vi "TomScan1762WithPumpingHWT.vi"() -> ()   [LabVIEW 2012]
uses:
  <vilib>/Utility/file.llb/Write To Spreadsheet File (DBL).vi
panel:
  out "OP Waveform":digitalwaveform(waveform)={"t0"=timestamp(0 s since 1904-01-01), "dt"=0.0, "Y"={"transitions"=[], "data"=[]}, "error"={"status"=FALSE, "code"=37421928, "source"=""}}
  in  "Comment":string="SPAOM, 3000 mA, 60 mA, 150 mA, now being mixed with 20 MHz, 7V Res, 89 MHz DPAOM"
  in  "B Field":dbl=3.0
  in  "Power":dbl=4.0
  out "digital waveform":digitalwaveform(waveform)={"t0"=timestamp(0 s since 1904-01-01), "dt"=0.001, "Y"={"transitions"=[], "data"=array3001x1[3001 elements]}}
  in  "Real Cutoff":dbl=26.0
  in  "Microseconds Expose":i32=300
  out "Shelving Events":dbl=11.0
  out "Dark Counts":dbl=19.0
  out "Bright Counts":dbl=61.0
  in  "Rerun BG":dbl=50.0
  in  "Interval":dbl=0.03
  in  "Runs for Background":dbl=50.0
  out "Average counts":dbl=59.98
  out "Cutoff":dbl=26.0
  in  "Cutoff Limit":dbl=10.0
  in  "OP Time":dbl=10.0
  in  "Op Pump":bool=TRUE
  in  "Runs per data point":dbl=100.0
  in  "Step Size":dbl(slide)=2000.0 min=100.0 max=100000.0 step=1.0 scale=100.0..100000.0 scale format="%#.0f"
  in  "Low Freq":dbl(slide)=78950000.0 min=50000000.0 max=120000000.0 step=1000.0 scale=50000000.0..120000000.0 scale format="%#.5f"
  in  "High Freq":dbl(slide)=79060000.0 min=50000000.0 max=120000000.0 step=1000.0 scale=50000000.0..120000000.0 scale format="%#.0f"
  out "Cur Freq":dbl=78998000.0 format="%#_8f"
  out "Path":path=path "c:/data/1762 Scans/2009-11-09_16-22-05_1762scanWithPumping.txt"
  out "Frequency Scan":cluster{dbl, dbl}[](graph)=[{79100000.0, 0.0}, {79098000.0, 0.01}, {79096000.0, 0.0}, {79094000.0, 0.0}, {79092000.0, 0.0}, {79090000.0, 0.01}, {79088000.0, 0.0}, {79086000.0, 0.0}, {79084000.0, 0.0}, {79082000.0, 0.0}, {79080000.0, 0.0}, {79078000.0, 0.0}, {79076000.0, 0.0}, {79074000.0, 0.02}, {79072000.0, 0.0}, {79070000.0, 0.0}, {79068000.0, 0.0}, {79066000.0, 0.0}, {79064000.0, 0.01}, {79062000.0, 0.0}, {79060000.0, 0.0}, {79058000.0, 0.02}, {79056000.0, 0.01}, {79054000.0, 0.01}, {79052000.0, 0.02}, {79050000.0, 0.01}, {79048000.0, 0.01}, {79046000.0, 0.05}, {79044000.0, 0.01}, {79042000.0, 0.01}, {79040000.0, 0.04}, {79038000.0, 0.02}, {79036000.0, 0.07}, {79034000.0, 0.07}, {79032000.0, 0.04}, {79030000.0, 0.08}, {79028000.0, 0.16}, {79026000.0, 0.22}, {79024000.0, 0.27}, {79022000.0, 0.31}, {79020000.0, 0.37}, {79018000.0, 0.49}, {79016000.0, 0.44}, {79014000.0, 0.36}, {79012000.0, 0.37}, {79010000.0, 0.48}, {79008000.0, 0.23}, {79006000.0, 0.29}, {79004000.0, 0.02}, {79002000.0, 0.02}, {79000000.0, 0.11}]
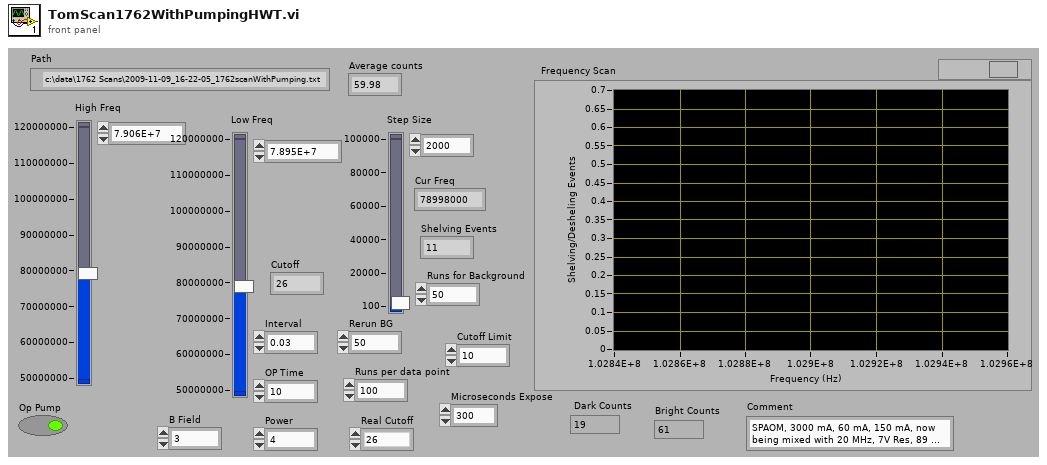
[diagram p1: front panel]
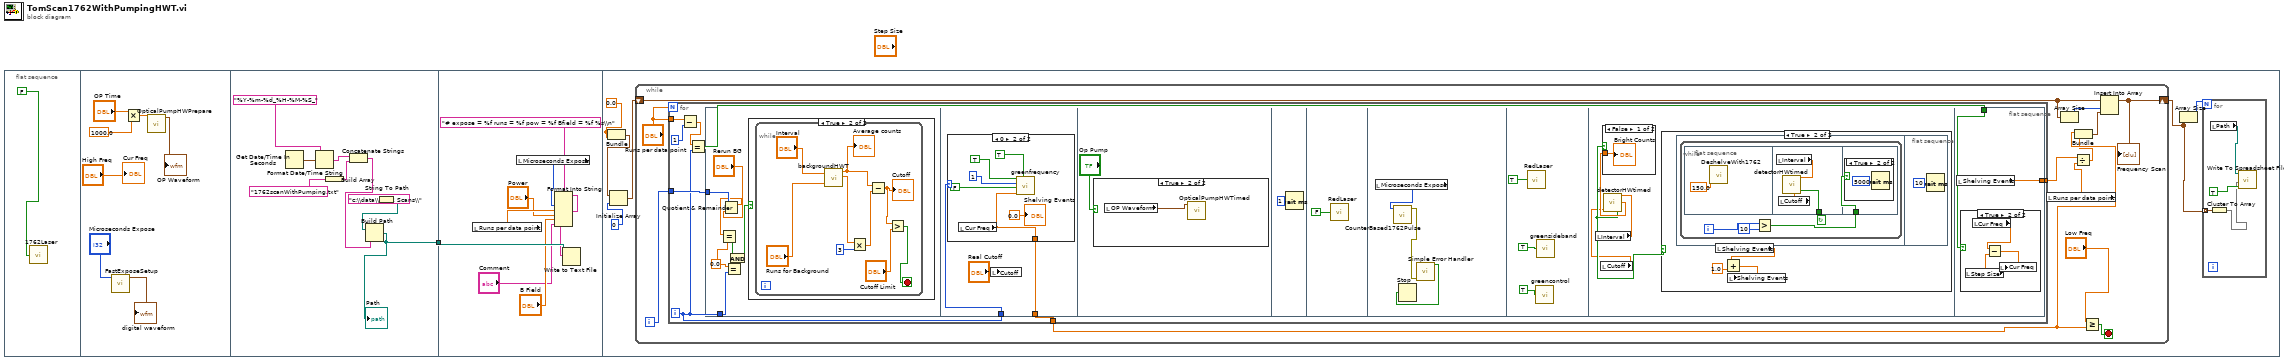
[diagram p0: block diagram]
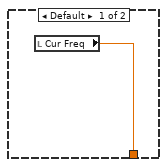
[diagram p3: hidden frame]
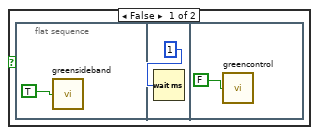
[diagram p4: hidden frame]
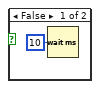
[diagram p6: hidden frame]
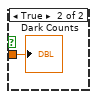
[diagram p7: hidden frame]
diagram:
  n1 = flat-sequence {
    tunnel: [w10] -> w1
    tunnel: w1 -> [w26]
    frame #0 {
      n2 = call "1762Laser.vi"("1762 Laser"=FALSE) -> ()
    }
    frame #1 {
      n3 = call "FastExposeSetup.vi"("Microseconds Expose"="Microseconds Expose") -> ("digital waveform"=→"digital waveform":digitalwaveform)  [unwired: 10 in]
      n4 = Multiply(x="OP Time", y=1000.0) -> (x*y=w4:dbl)
      n5 = call "OpticalPumpHWPrepare.vi"("Pump Expose Time (us)"=w4) -> ("digital waveform out"=→"OP Waveform":digitalwaveform)  [unwired: 8 in]
      "Cur Freq" <- "High Freq"
    }
    frame #2 {
      n6 = Get Date/Time In Seconds() -> (seconds since 1Jan1904=w12:timestamp)
      n7 = Format Date/Time String(time format string (%c)="%Y-%m-%d_%H-%M-%S_", seconds (now)=w12) -> (date/time string=w14:string)  [unwired: 1 in]
      n8 = Build Array("1762scanWithPumping.txt") -> (w17:string[])
      n9 = Concatenate Strings(w14, w17) -> (w16:string)
      n10 = String To Path(string="c:\\data\\1762 Scans\\") -> (path=w18:path)
      n11 = Build Path(base path=w18, name or relative path=w16) -> (appended path=w10:path)
      "Path" <- w10
    }
    frame #3 {
      n12 = local read "Runs per data point"() -> (w22:dbl)
      n13 = local read "Microseconds Expose"() -> (w23:i32)
      n14 = Format Into String(format string="# expose = %f runs = %f pow = %f Bfield = %f %s\\n", w23, w22, "Power", "B Field", "Comment") -> (resulting string=w24:string)  [unwired: 2 in, 1 out]
      n15 = Write to Text File(file (use dialog)=w26, text=w24) -> ()  [unwired: 2 in, 3 out]
    }
    frame #4 {
      w31 = 0.0
      n16 = Bundle(w31, w31) -> (w32:cluster{dbl, dbl})  [unwired: 1 in]
      n17 = Initialize Array(w32, 0) -> (w29:cluster{dbl, dbl}[])
      n18 = while {
        shift-right: [w40] -> w27
        shift-left: w29 -> [w41]
        i -> [w48]
        stop <- w46 stop-if-true
        n19 = for {
          N: "Runs per data point" -> [_]
          tunnel: w48 -> [w56]
          tunnel: [w55] -> w38
          tunnel: [w54] -> w45
          tunnel: "Runs per data point" -> [w49]
          i -> [w53]
          n20 = Subtract(x=w49, y=1) -> (x-y=w52:dbl)
          n21 = Equal?(x=w52, y=w53) -> (x = y?=w50:bool)
          n22 = flat-sequence {
            tunnel: w53 -> [w64]
            tunnel: w56 -> [w63]
            tunnel: w53 -> [w76]
            tunnel: [w75] -> w55
            tunnel: [w119] -> w54
            tunnel: w50 -> [w118]
            frame #0 {
              w60 = 0.0 ("x")
              n23 = Quotient & Remainder(x=w63, y="Rerun BG") -> (x-y*floor(x/y)=w61:dbl)  [unwired: 1 out]
              n24 = Equal?(x=w61, y=w60) -> (x = y?=w58:bool)
              n25 = Equal?(x=w60, y=w64) -> (x = y?=w59:bool)
              n26 = And(x=w58, y=w59) -> (x .and. y?=w57:bool)
              n27 = case shown="True" w57 {
                frame False {
                }
                frame True {
                  n28 = while {
                    stop <- w65 stop-if-true
                    n29 = call "backgroundHWT.vi"("Interval"="Interval", "Runs"="Runs for Background") -> ("Mean"=w72:dbl, "Deviation"=w71:dbl)  [unwired: 2 out]
                    "Average counts" <- w72
                    n30 = Multiply(x=w71, y=3) -> (x*y=w73:dbl)
                    n31 = Subtract(x=w72, y=w73) -> (x-y=w67:dbl)
                    "Cutoff" <- w67
                    n32 = Greater?(x=w67, y="Cutoff Limit") -> (0:w65:bool)
                  }
                }
              }
            }
            frame #1 {
              n33 = case shown="0" w76 {
                tunnel: [w77 w79] -> w75
                frame Default {
                  n34 = local read "Cur Freq"() -> (w77:dbl)
                }
                frame 0 {
                  n35 = local read "Cur Freq"() -> (w79:dbl)
                  n36 = call "greenfrequency.vi"("Send Frequency"=TRUE, "Level"=1, "Send Level"=FALSE, "Frequency"=w79, "Stop"=TRUE) -> ()  [unwired: 2 in]
                  "Shelving Events" <- 0.0 ("Shelving Events")
                }
              }
              n37 = local write "Cutoff"("Real Cutoff") -> ()
            }
            frame #2 {
              n38 = case shown="True" "Op Pump" {
                frame False {
                  n39 = flat-sequence {
                    frame #0 {
                      n40 = call "greensideband.vi"("Sideband On/Off"=TRUE) -> ()
                    }
                    frame #1 {
                      n41 = Wait (ms)(milliseconds to wait=1) -> ()  [unwired: 1 out]
                    }
                    frame #2 {
                      n42 = call "greencontrol.vi"("Green"=FALSE) -> ()
                    }
                  }
                }
                frame True {
                  n43 = local read "OP Waveform"() -> (w88:digitalwaveform)
                  n44 = call "OpticalPumpHWTimed.vi"("OP Waveform"=w88) -> ()  [unwired: 10 in, 1 out]
                }
              }
            }
            frame #3 {
              n45 = Wait (ms)(milliseconds to wait=u32 1) -> ()  [unwired: 1 out]
            }
            frame #4 {
              n46 = call "RedLaser.vi"("Red Laser"=FALSE) -> ()
            }
            frame #5 {
              n47 = local read "Microseconds Expose"() -> (w91:i32)
              n48 = call "CounterBased1762Pulse.vi"("High Time (us)"=w91) -> ("error out"=w92:errorcluster)  [unwired: 10 in]
              n49 = call <vilib>:"Simple Error Handler.vi"("error in (no error)"=w92) -> ("error?"=w93:bool)  [unwired: 4 in, 4 out]
              n50 = Stop(stop? (T)=w93) -> ()
            }
            frame #6 {
              n51 = call "RedLaser.vi"("Red Laser"=TRUE) -> ()
              n52 = call "greencontrol.vi"("Green"=TRUE) -> ()
              n53 = call "greensideband.vi"("Sideband On/Off"=TRUE) -> ()
            }
            frame #7 {
              n54 = local read "Interval"() -> (w99:dbl)
              n55 = local read "Cutoff"() -> (w97:dbl)
              n56 = call "detectorHWtimed.vi"("Cutoff"=w97, "Interval"=w99) -> ("Boolean"=w98:bool, "Counts"=w100:dbl)  [unwired: 3 in]
              n57 = case shown="False" w98 {
                tunnel: w100 -> [w116 w117]
                frame False {
                  "Bright Counts" <- w116
                }
                frame True {
                  "Dark Counts" <- w117
                }
              }
              n58 = case shown="True" w98 {
                frame False {
                }
                frame True {
                  n59 = flat-sequence {
                    frame #0 {
                      n60 = while {
                        i -> [w106]
                        stop <- w107 continue-if-true
                        n61 = flat-sequence {
                          tunnel: [w109] -> w107
                          tunnel: w104 -> [w112]
                          frame #0 {
                            n62 = call "DeshelveWith1762.vi"("Expose Time"=150.0) -> ()
                          }
                          frame #1 {
                            n63 = local read "Interval"() -> (w111:dbl)
                            n64 = local read "Cutoff"() -> (w110:dbl)
                            n65 = call "detectorHWtimed.vi"("Cutoff"=w110, "Interval"=w111) -> ("Boolean"=w109:bool)  [unwired: 3 in, 1 out]
                          }
                          frame #2 {
                            n66 = case shown="True" w112 {
                              frame False {
                                n67 = Wait (ms)(milliseconds to wait=u32 10) -> ()  [unwired: 1 out]
                              }
                              frame True {
                                n68 = Wait (ms)(milliseconds to wait=u32 5000) -> ()  [unwired: 1 out]
                              }
                            }
                          }
                        }
                        n69 = Greater?(x=w106, y=10) -> (0:w104:bool)
                      }
                    }
                    frame #1 {
                      n70 = Wait (ms)(milliseconds to wait=u32 10) -> ()  [unwired: 1 out]
                    }
                  }
                  n71 = local read "Shelving Events"() -> (w102:dbl)
                  n72 = Add(x=w102, y=1.0) -> (x+y=w101:dbl)
                  n73 = local write "Shelving Events"(w101) -> ()
                }
              }
            }
            frame #8 {
              n74 = local read "Shelving Events"() -> (w119:dbl)
              n75 = case shown="True" w118 {
                frame False {
                }
                frame True {
                  n76 = local read "Step Size"() -> (w121:dbl)
                  n77 = local read "Cur Freq"() -> (w122:dbl)
                  n78 = Subtract(x=w122, y=w121) -> (x-y=w120:dbl)
                  n79 = local write "Cur Freq"(w120) -> ()
                }
              }
            }
          }
        }
        n80 = local read "Runs per data point"() -> (w44:dbl)
        n81 = Array Size(array=w41) -> (size(s)=w43:i32)
        n82 = Divide(x=w45, y=w44) -> (x/y=w37:dbl)
        n83 = Bundle("Cur Freq"=w38, w37) -> (w42:cluster{"Cur Freq":dbl, dbl})  [unwired: 1 in]
        n84 = Greater Or Equal?(x="Low Freq", y=w38) -> (x >= y?=w46:bool)
        n85 = Insert Into Array(array=w41, index=w43, new element=w42) -> (w40:cluster{dbl, dbl}[])
        "Frequency Scan" <- w40
      }
      n86 = Array Size(array=w27) -> (size(s)=w28:i32)
      n87 = for {
        N: w28 -> [_]
        tunnel: w27 -> [w36] mode=indexing
        n88 = local read "Path"() -> (w33:path)
        n89 = Cluster To Array(cluster=w36) -> (array=w34:dbl[])
        n90 = call-poly <vilib>:"Write To Spreadsheet File.vi"("append to file? (new file:F)"=TRUE, "1D data"=w34, "file path (dialog if empty)"=w33) -> ()  [unwired: 5 in, 1 out]
      }
    }
  }
